vi "Write DI_reorder_table.vi"(8 "error in (no error)":errorcluster, 10 "OPC UA client refnum in":T1, 11 "EnumsDI":string[](array[string])) -> (0 "error out":errorcluster, 2 "connect":bool, 3 "DI_reorder_table":i32[](array[numeric]))   [LabVIEW 2019, in "OPC addons.lvlib"]
uses:
  <vilib>/OPCUA/controls/OPC UA Client Refnum.ctl
  <vilib>/OPCUA/controls/NodeIds.ctl
  <vilib>/OPCUA/controls/NodeId.ctl
  <vilib>/OPCUA/client/Multiple Read String Array.vi
  OPC addons.lvlib
  <vilib>/OPCUA/NI OPC UA Client.lvlib
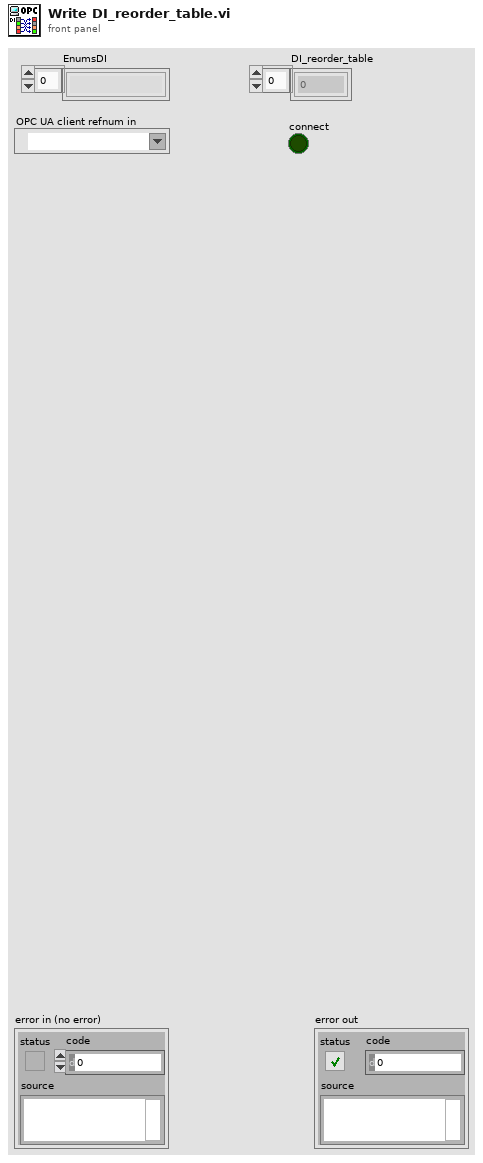
[diagram p1: front panel]
types:
  T1 = typedef "OPC UA Client Refnum.ctl" = refnum<k21>
  T2 = typedef "NodeIds.ctl" = T3[]
  T3 = typedef "NodeId.ctl" = string
  T4 = typedef "OPC UA StatusCode.ctl" = u32
  T5 = cluster{"node ID":T3, "values ":string[], "timestamp":timestamp, "status":T4}[]
  T6 = cluster{"node ID":T3, "values ":string[], "timestamp":timestamp, "status":T4}
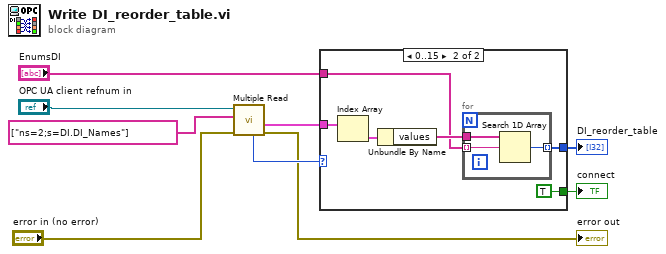
[diagram p0: block diagram]
diagram:
  n1 = call-poly <vilib>:"Multiple Read.vi"("error in (no error)"="error in (no error)", "node IDs"=T2 ["ns=2;s=DI.DI_Names"] ("OPC UA.node IDs"), "OPC UA client refnum in"="OPC UA client refnum in") -> ("error out"=→"error out":errorcluster, "results"=w9:T5, "service status"=w8:T4)  [unwired: 5 in, 1 out]
  n2 = case shown="0..15" w8 {
    tunnel: w9 -> [_ w14]
    tunnel: "EnumsDI" -> [_ w12]
    tunnel: [_ w11] -> w6
    tunnel: [_ TRUE] -> w4
    frame 16.., Default {
    }
    frame 0..15 {
      n3 = Index Array(array=w14) -> (element=w15:T6)  [unwired: 1 in]
      n4 = Unbundle By Name(w15) -> ("values"=w13:string[])
      n5 = for {
        tunnel: w12 -> [w18] mode=indexing
        tunnel: w13 -> [w17]
        tunnel: [w16] -> w11 mode=indexing
        n6 = Search 1D Array(1D array=w17, element=w18) -> (index of element=w16:i32)  [unwired: 1 in]
      }
    }
  }
  "connect" <- w4
  "DI_reorder_table" <- w6
